vi "FPGA PWM.vi"(7 "PWM Enabled?":bool, 9 "Duty Cycle (0-100)":i8, 10 "Desired PWM Frequency (Hz)":i32, 11 "Source Frequency (Hz)":i32) -> (2 "PWM Exact?":bool, 3 "PWM Output":bool)   [LabVIEW 2014]
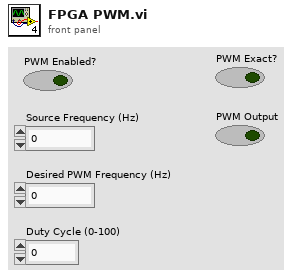
[diagram p1: front panel]
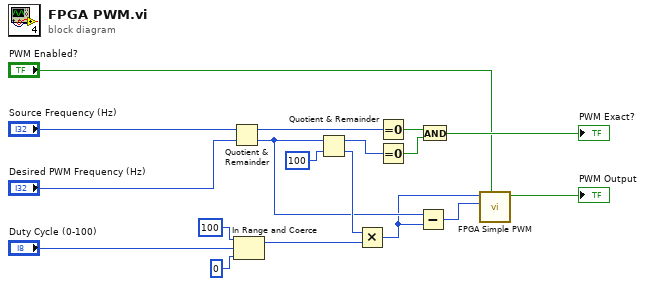
[diagram p0: block diagram]
diagram:
  n1 = Quotient & Remainder(x="Source Frequency (Hz)", y="Desired PWM Frequency (Hz)") -> (x-y*floor(x/y)=w4:i32, floor(x/y)=w12:i32)
  n2 = In Range and Coerce(upper limit=i8 100, x="Duty Cycle (0-100)", lower limit=i8 0 ("upper limit")) -> (coerced(x)=w7:i8)  [unwired: 1 out]
  n3 = Quotient & Remainder(x=w12, y=100) -> (x-y*floor(x/y)=w1:i32, floor(x/y)=w13:i32)
  n4 = Multiply(x=w13, y=w7) -> (x*y=w10:i32)
  n5 = Equal To 0?(x=w4) -> (x = 0?=w15:bool)
  n6 = Equal To 0?(x=w1) -> (x = 0?=w14:bool)
  n7 = Subtract(x=w12, y=w10) -> (x-y=w11:i32)
  n8 = And(x=w15, y=w14) -> (x .and. y?=→"PWM Exact?":bool)
  n9 = call "FPGA Simple PWM.vi"("PWM Enabled?"="PWM Enabled?", "Low Ticks"=w11, "High Ticks"=w10) -> ("PWM Output"=→"PWM Output":bool)  [unwired: 8 in]
